vi "Level.vi"(11 "DataIn":T4) -> (3 "Cluster":T1)   [LabVIEW 2017]
uses:
  controls/DataIn.ctl
  controls/Tabuleiro.ctl
  controls/GameOption.ctl
  controls/DataOut.ctl
panel:
  in  "Médio":bool
  in  "Fácil":bool
  # "Escolha a dificuldade"
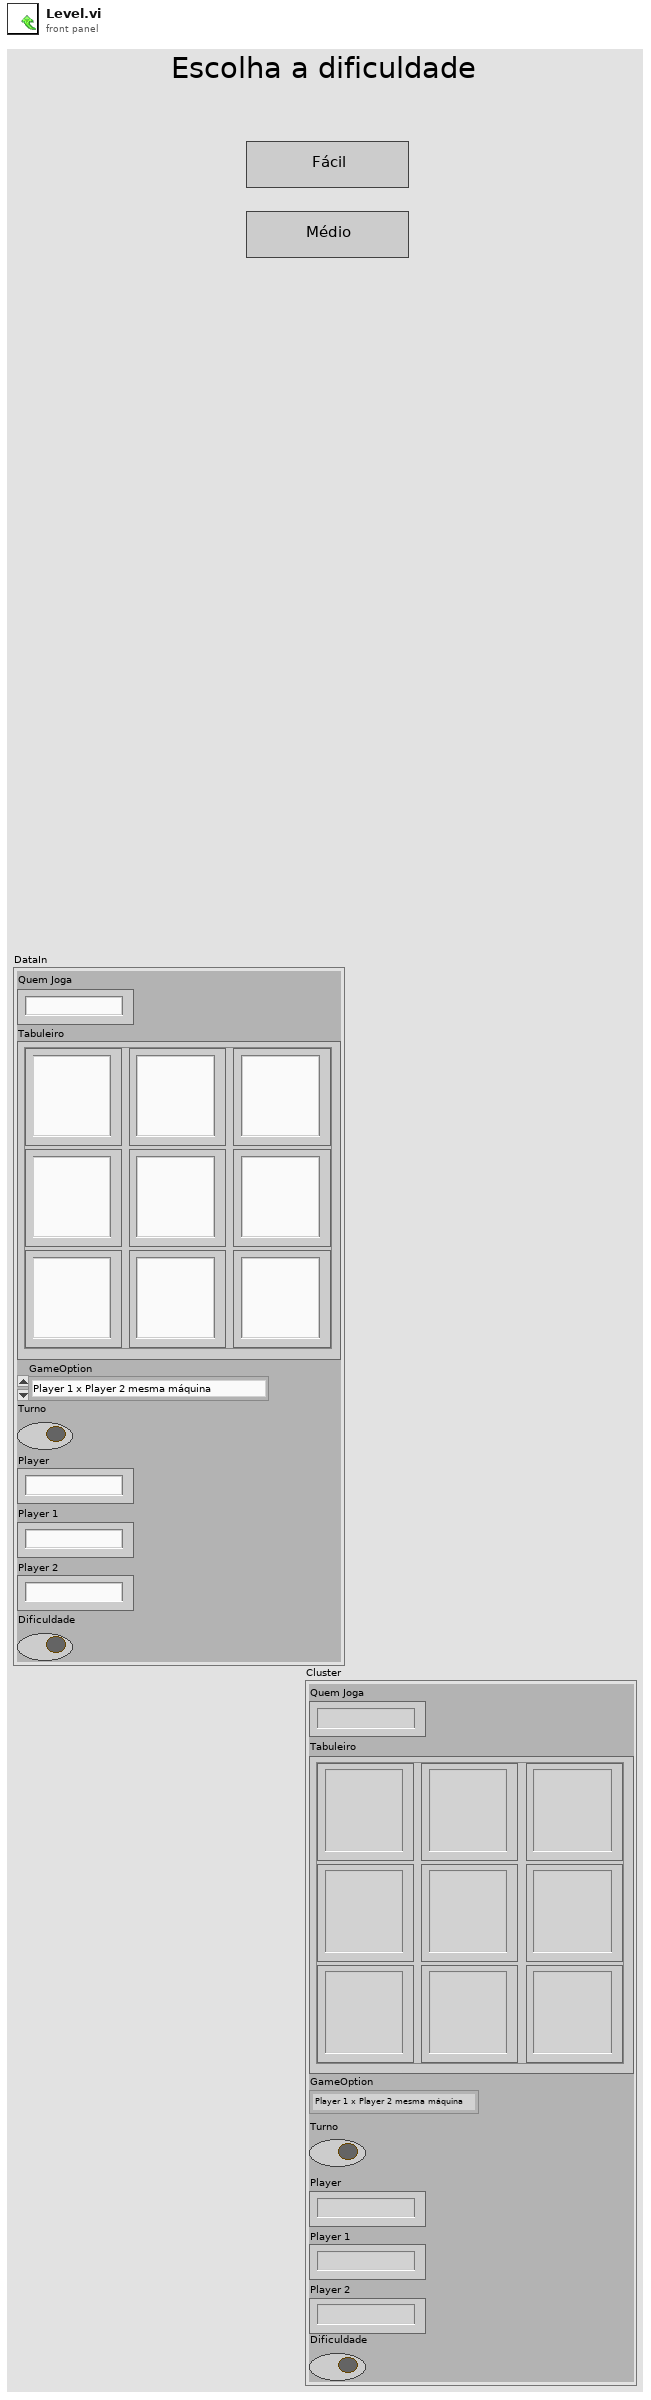
[diagram p1: front panel]
types:
  T1 = typedef "DataOut.ctl" = cluster{"Quem Joga":string, "Tabuleiro":T2, "GameOption":T3, "Turno":bool, "Player":string, "Player 1":string, "Player 2":string, "Dificuldade":bool}
  T2 = typedef "Tabuleiro.ctl" = cluster{"(0,0)":string, "(1,0)":string, "(0,1)":string, "(1,1)":string, "(2,0)":string, "(1,2)":string, "(2,2)":string, "(0,2)":string, "(2,1) ":string}
  T3 = typedef "GameOption.ctl" = enum16{"Player 1 x Player 2 mesma máquina", "Player 1 x Player 2 pela rede", "Player 1 x Computador", "Wait for Event", "Initialize"}
  T4 = typedef "DataIn.ctl" = cluster{"Quem Joga":string, "Tabuleiro":T2, "GameOption":T3, "Turno":bool, "Player":string, "Player 1":string, "Player 2":string, "Dificuldade":bool}
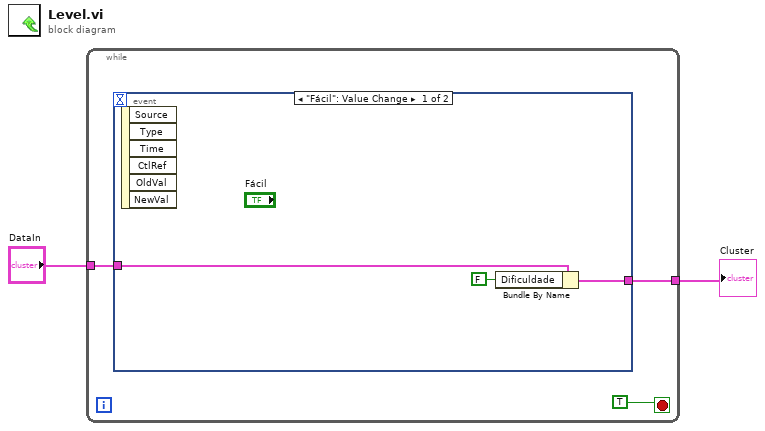
[diagram p0: block diagram]
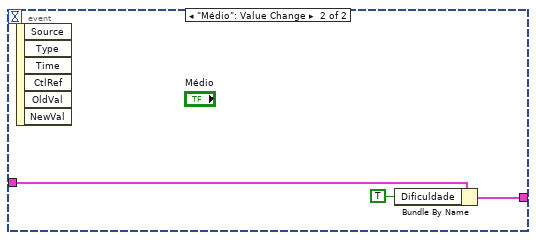
[diagram p2: hidden frame]
diagram:
  n1 = while {
    tunnel: "DataIn" -> [w5]
    tunnel: [w3] -> w1
    stop <- TRUE stop-if-true
    n2 = event shown="[0] \"Fácil\": Value Change" {
      selector: _ -> [_ _]
      dyn-events: _ -> [_ _]
      timeout: _ -> [_ _]
      tunnel: w5 -> [w7 w10]
      tunnel: [w8 w11] -> w3
      event "Fácil": Value Change {
        n3 = event-data() -> ()  [unwired: 1 in, 6 out]
        n4 = Bundle By Name(cluster=w7, "Dificuldade"=FALSE) -> (w8:T4)
      }
      event "Médio": Value Change {
        n5 = event-data() -> ()  [unwired: 1 in, 6 out]
        n6 = Bundle By Name(cluster=w10, "Dificuldade"=TRUE) -> (w11:T4)
      }
    }
  }
  "Cluster" <- w1
